vi "VI Tree.vi"   [LabVIEW 2016, in "Error Manager.lvlib" / "Error Log.lvclass"]
doc: "VI Tree\nThis VI lists all the public VIs and CTLs of the library."
uses:
  Error Log.lvclass
  Error Type (enum).ctl
  Error to be logged (cluster).ctl
panel:
  # "VI Tree\nSee the block diagram for the VI Tree"
types:
  T1 = typedef "Error Manager.lvlib/Error Log.lvclass/Error to be logged (cluster).ctl" = cluster{"Error Type":T2, "Error Number":i32, "Error Timestamp":timestamp, "Error code":i32, "Error message":string}
  T2 = typedef "Error Manager.lvlib/Error Log.lvclass/Error Type (enum).ctl" = enum16{"New", "Identical to last logged error"}
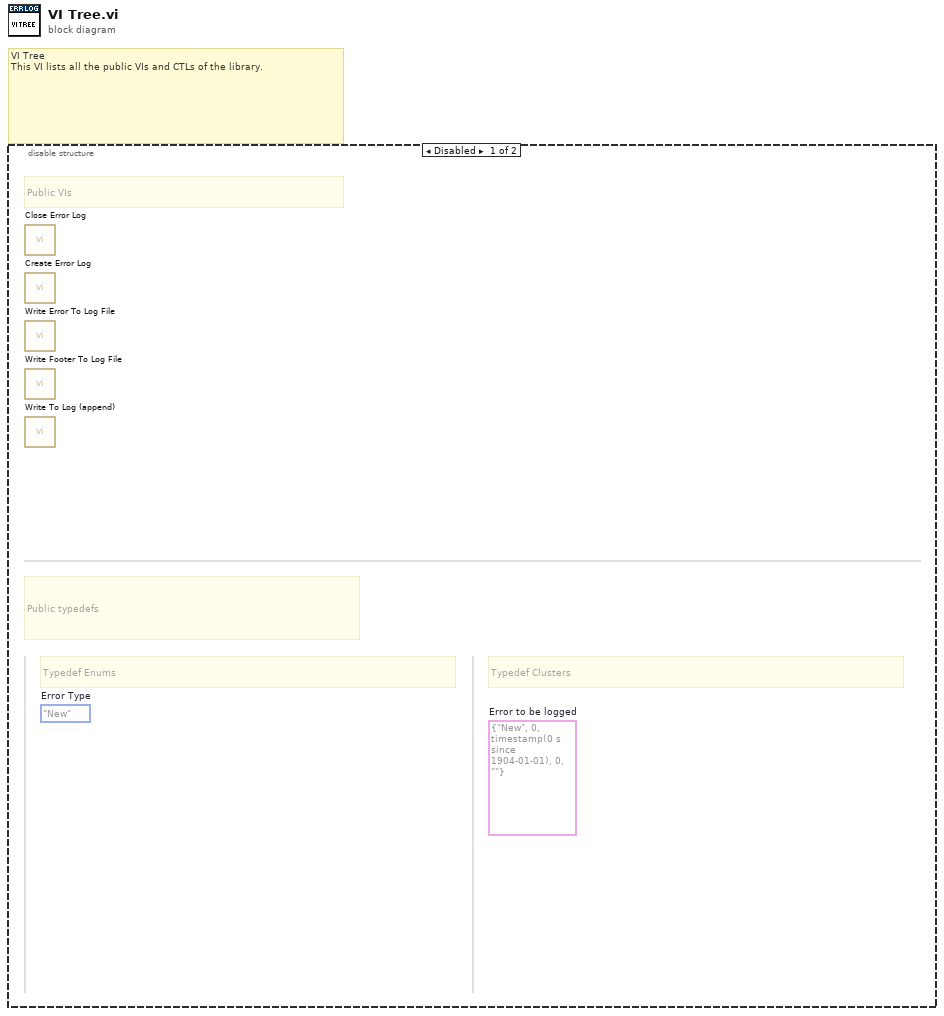
[diagram p0: block diagram]
diagram:
  # "VI Tree\nThis VI lists all the public VIs and CTLs of the library."
  n1 = disable-structure shown="Disabled" {
    frame Disabled {
      (unwired) T1 {"Error Type"=enum."New", "Error Number"=0, "Error Timestamp"=timestamp(0 s since 1904-01-01), "Error code"=0, "Error message"=""}  # Error to be logged
      (unwired) Error_Type_(enum)."New"  # Error Type
      # "Typedef Clusters"
      # "Typedef Enums"
      # "Public typedefs"
      # "Public VIs"
      n2 = call "Close Error Log.vi"() -> ()  [unwired: 11 in, 1 out]
      n3 = call "Create Error Log.vi"() -> ()  [unwired: 10 in, 2 out]
      n4 = call "Write Error To Log File.vi"() -> ()  [unwired: 11 in, 1 out]
      n5 = call "Write Footer To Log File.vi"() -> ()  [unwired: 11 in, 1 out]
      n6 = call "Write To Log (append).vi"() -> ()  [unwired: 11 in, 1 out]
    }
    frame Enabled {
    }
  }
